vi "serial_06.vi"(0 "VISA resource name":refnum<visa-resource-name>="COM4") -> ()   [LabVIEW 2010]
doc: "The Basic Serial Read and Write example performs a Serial Port Read, a Serial Port Write, or a combination of these actions. The user selects the actions (read or write) on the front panel. If both are selected, the VI will write the data first, read data, and then close the VISA session that is opened to the port. This VI will wait until the specified number of bytes is received at the port. Only the number of bytes specified will be read.\n\nINSTRUCTIONS:\n1) Select the serial resource and configuration parameters (baud rate, data bits, parity, stop bits, flow control).\n2) Select the operations to be performed. \n3) Connect the serial port to your device. If no device is available, perform a loopback test by doing one of the following. Short pins 2 and 3 on a RS-232 cable or short pin 4 to pin 8 and pin 5 to pin 9 on a RS-485/422 cable. \n4) Run the VI to see the data read. (The \"read string\" will match the \"string to write\" if a loopback test was performed.)\n\nNote: The parameters set for the serial port must match the parameters of the connected instrument or device. In this example, the bytes to read parameter specifies the number of bytes that the serial port reads. If there were more bytes at the port than the number specified in bytes to read, those bytes would not be read. Also, if you specify to read more bytes than the number of bytes actually read, you might receive a timeout error message.\n\nOn the block diagram, the Configure Serial Port VI sets the configuration parameters. The front panel displays the controls used to configure the basic parameters, such as baud rate, data bits, and parity. Constants configure the other parameters the user probably does not need set. After the VISA Configure Serial Port VI opens the VISA session and configures the port, the VI passes the VISA resource name to other VIs that perform operations on that VISA resource. The VISA Write function sends a command to the serial device and the VISA Read function returns data based on the command. The VISA Close function then closes the reference to the serial device. It is important to close the reference; otherwise communication through with that port through protocols other than VISA might not be possible."
panel:
  out "A4":dbl(knob) scale=0.0..1024.0
  out "A3":dbl(knob) scale=0.0..1024.0
  out "A2":dbl(knob) scale=0.0..1024.0
  out "A1":dbl(knob) scale=0.0..1024.0
  out "A0":dbl(knob) scale=0.0..1024.0
  out "A4":string
  out "A3":string
  out "A2":string
  out "A1":string
  out "A0":string
  out "String":string
  in  "Start":bool=TRUE
  # "Stop"
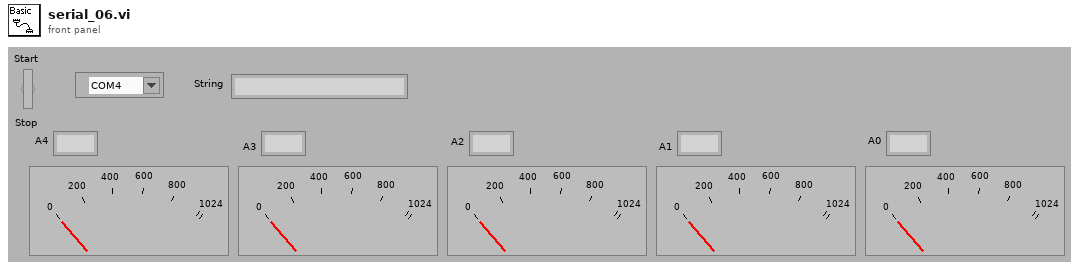
[diagram p1: front panel]
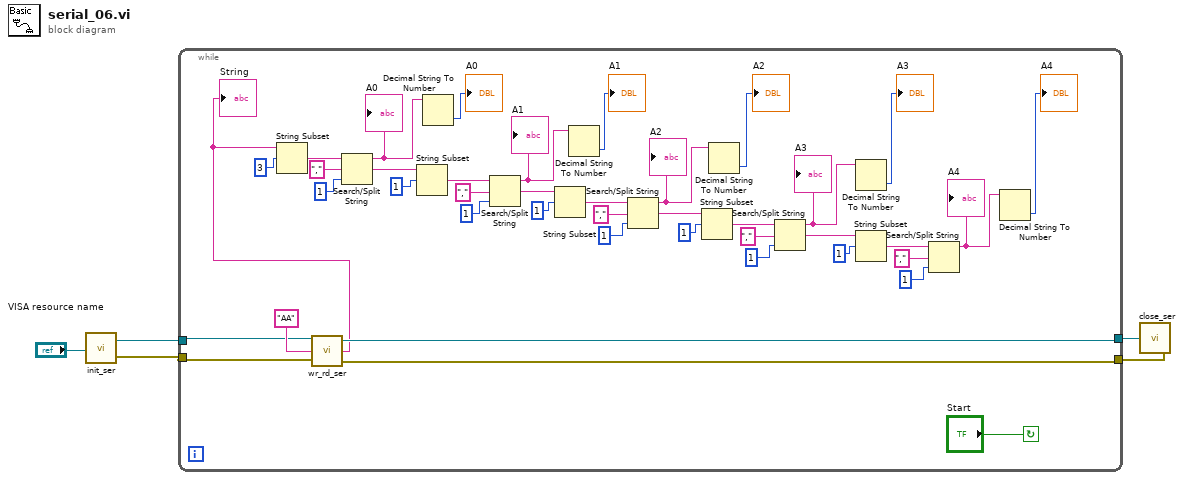
[diagram p0: block diagram]
diagram:
  n1 = call "init_ser.vi"("VISA resource name"="VISA resource name") -> ("VISA resource name out"=w3:refnum<visa-resource-name>, "error out"=w4:errorcluster)
  n2 = while {
    tunnel: w4 -> [w11]
    tunnel: w3 -> [w12]
    tunnel: [w43] -> w2
    tunnel: [w44] -> w1
    stop <- "Start" continue-if-true
    n3 = call "wr_rd_ser.vi"("error in"=w11, "string to write"="AA", "VISA resource name in"=w12) -> ("error out"=w43:errorcluster, "read buffer"=w34:string, "VISA resource name out"=w44:refnum<visa-resource-name>)
    "String" <- w34
    n4 = String Subset(string=w34, offset (0)=3) -> (substring=w33:string)  [unwired: 1 in]
    n5 = Search/Split String(string=w33, search string/char (-)=",", offset (0)=1) -> (substring before match=w17:string, match + rest of string=w38:string)  [unwired: 1 out]
    "A0" <- w17
    n6 = String Subset(string=w38, offset (0)=1) -> (substring=w36:string)  [unwired: 1 in]
    n7 = Decimal String To Number(string=w17) -> (number=→"A0":i32)  [unwired: 2 in, 1 out]
    n8 = Search/Split String(string=w36, search string/char (-)=",", offset (0)=1 ("x")) -> (substring before match=w16:string, match + rest of string=w28:string)  [unwired: 1 out]
    "A1" <- w16
    n9 = String Subset(string=w28, offset (0)=1) -> (substring=w29:string)  [unwired: 1 in]
    n10 = Decimal String To Number(string=w16) -> (number=→"A1":i32)  [unwired: 2 in, 1 out]
    n11 = Search/Split String(string=w29, search string/char (-)=",", offset (0)=1 ("x")) -> (substring before match=w15:string, match + rest of string=w23:string)  [unwired: 1 out]
    "A2" <- w15
    n12 = String Subset(string=w23, offset (0)=1) -> (substring=w24:string)  [unwired: 1 in]
    n13 = Decimal String To Number(string=w15) -> (number=→"A2":i32)  [unwired: 2 in, 1 out]
    n14 = Search/Split String(string=w24, search string/char (-)=",", offset (0)=1 ("x")) -> (substring before match=w14:string, match + rest of string=w18:string)  [unwired: 1 out]
    "A3" <- w14
    n15 = Decimal String To Number(string=w14) -> (number=→"A3":i32)  [unwired: 2 in, 1 out]
    n16 = String Subset(string=w18, offset (0)=1) -> (substring=w19:string)  [unwired: 1 in]
    n17 = Search/Split String(string=w19, search string/char (-)=",", offset (0)=1 ("x")) -> (substring before match=w13:string)  [unwired: 2 out]
    "A4" <- w13
    n18 = Decimal String To Number(string=w13) -> (number=→"A4":i32)  [unwired: 2 in, 1 out]
  }
  n19 = call "close_ser.vi"("error in"=w2, "VISA resource name in"=w1) -> ()
